vi "PBPCIcard_suspend.vi"(2 "error in":errorcluster) -> (0 "error out":errorcluster)   [LabVIEW 2013]
uses:
  pbcomm32.vi
panel:
  in  "Base Address":u32 format="%.0x"
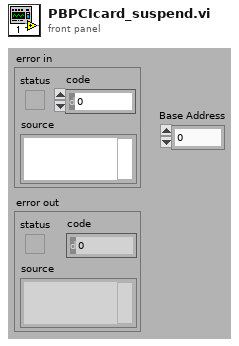
[diagram p1: front panel]
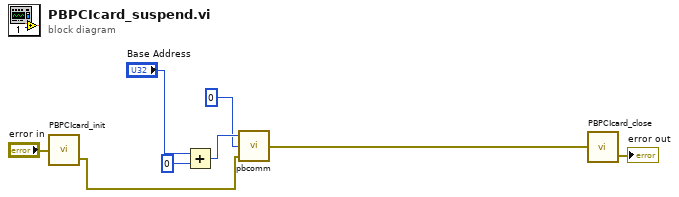
[diagram p0: block diagram]
diagram:
  n1 = call "PBPCIcard_init.vi"("error in"="error in") -> ("error out"=w4:errorcluster)  [unwired: 1 out]
  n2 = Add(x="Base Address", y=u32 0) -> (x+y=w5:u32)
  n3 = call-poly "pbcomm.vi"("error in"=w4, "write value"=0, "address"=w5) -> ("error out"=w1:errorcluster)
  n4 = call "PBPCIcard_close.vi"("error in"=w1) -> ("error out"=→"error out":errorcluster)  [unwired: 1 out]
